vi "PXI Loop Back.vi"() -> ()   [LabVIEW 2015]
uses:
  <vilib>/Platform/TimedLoop/XDataNode/wakeup.ctl
  <vilib>/Platform/TimedLoop/XDataNode/XDNodeRunTimeDep.lvlib
  <vilib>/Platform/TimedLoop/XDataNode/nitl_modes.ctl
  <vilib>/Platform/TimedLoop/XDataNode/timing_clust.ctl
  <vilib>/Platform/TimedLoop/XDataNode/XDataNode.xnode
  <vilib>/eio/EIONode/EIONode.xnode
  <vilib>/NI Veristand/FPGA/NI_VS FPGA Support.lvlib
  <vilib>/eio/EIOMethodNode/EIOMethodNode.xnode
  <vilib>/rvi/eio/common/nirviEmuTemplateMethod_errors.vi
panel:
  in  "Enable Line":bool
  in  "ENC 2 Direction":bool
  in  "ENC 2 Periods/tic":fxp<+,32,0> format="%.32g"
  in  "ENC 1 Direction":bool
  in  "ENC 1 Periods/tic":fxp<+,32,0> format="%.32g"
  in  "ENC 0 Periods/tic":fxp<+,32,0> format="%.32g"
  in  "ENC 0 Direction":bool
  out "ENC 2 In Velocity":i32
  out "ENC 2 In Position":i32
  out "ENC 2 In Vel/Acc Update":bool
  out "ENC 1 In Velocity":i32
  out "ENC 1 In Position":i32
  out "ENC 1 In Vel/Acc Update":bool
  out "ENC 0 In Velocity":i32
  out "ENC 0 In Position":i32
  out "ENC 0 In Vel/Acc Update":bool
  in  "ENC In Clock":bool=TRUE
  in  "PWM 3 Out Low Loopback":u32
  in  "PWM 3 Out High Loopback":u32
  in  "PWM 2 Out Low Loopback":u32
  in  "PWM 2 Out High Loopback":u32
  out "PWM 1 In Low Loopback":u32
  out "PWM 1 In High Loopback":u32
  in  "PWM 1 In Timeout Loopback":u32=40000
  out "PWM 0 In Low Loopback":u32
  out "PWM 0 In High Loopback":u32
  in  "PWM 0 In Timeout Loopback":u32=40000
  out "PWM 3 In Low Time":u32
  out "PWM 3 In High Time":u32
  in  "PWM 3 In Timeout":u32=40000
  out "PWM 2 In Low Time":u32
  out "PWM 2 In High Time":u32
  in  "PWM 2 In Timeout":u32=40000
  in  "PWM 1 Out Low Time":u32
  in  "PWM 1 Out High Time":u32
  in  "PWM 0 Out Low Time":u32
  in  "PWM 0 Out High Time":u32
  in  "Generate IRQ":bool
  in  "Clock Pulse":bool
  in  "Clock Ticked":bool
  in  "Use External Timing":bool
  in  "Write to  RTSI":bool
  in  "Loop Rate (usec)":u32
  in  "Start":bool
  # "PWM out"
  # "PWM In"
  # "Encoder in"
  # "Encoder out"
  # "Configuration"
  # "Internal Controls"
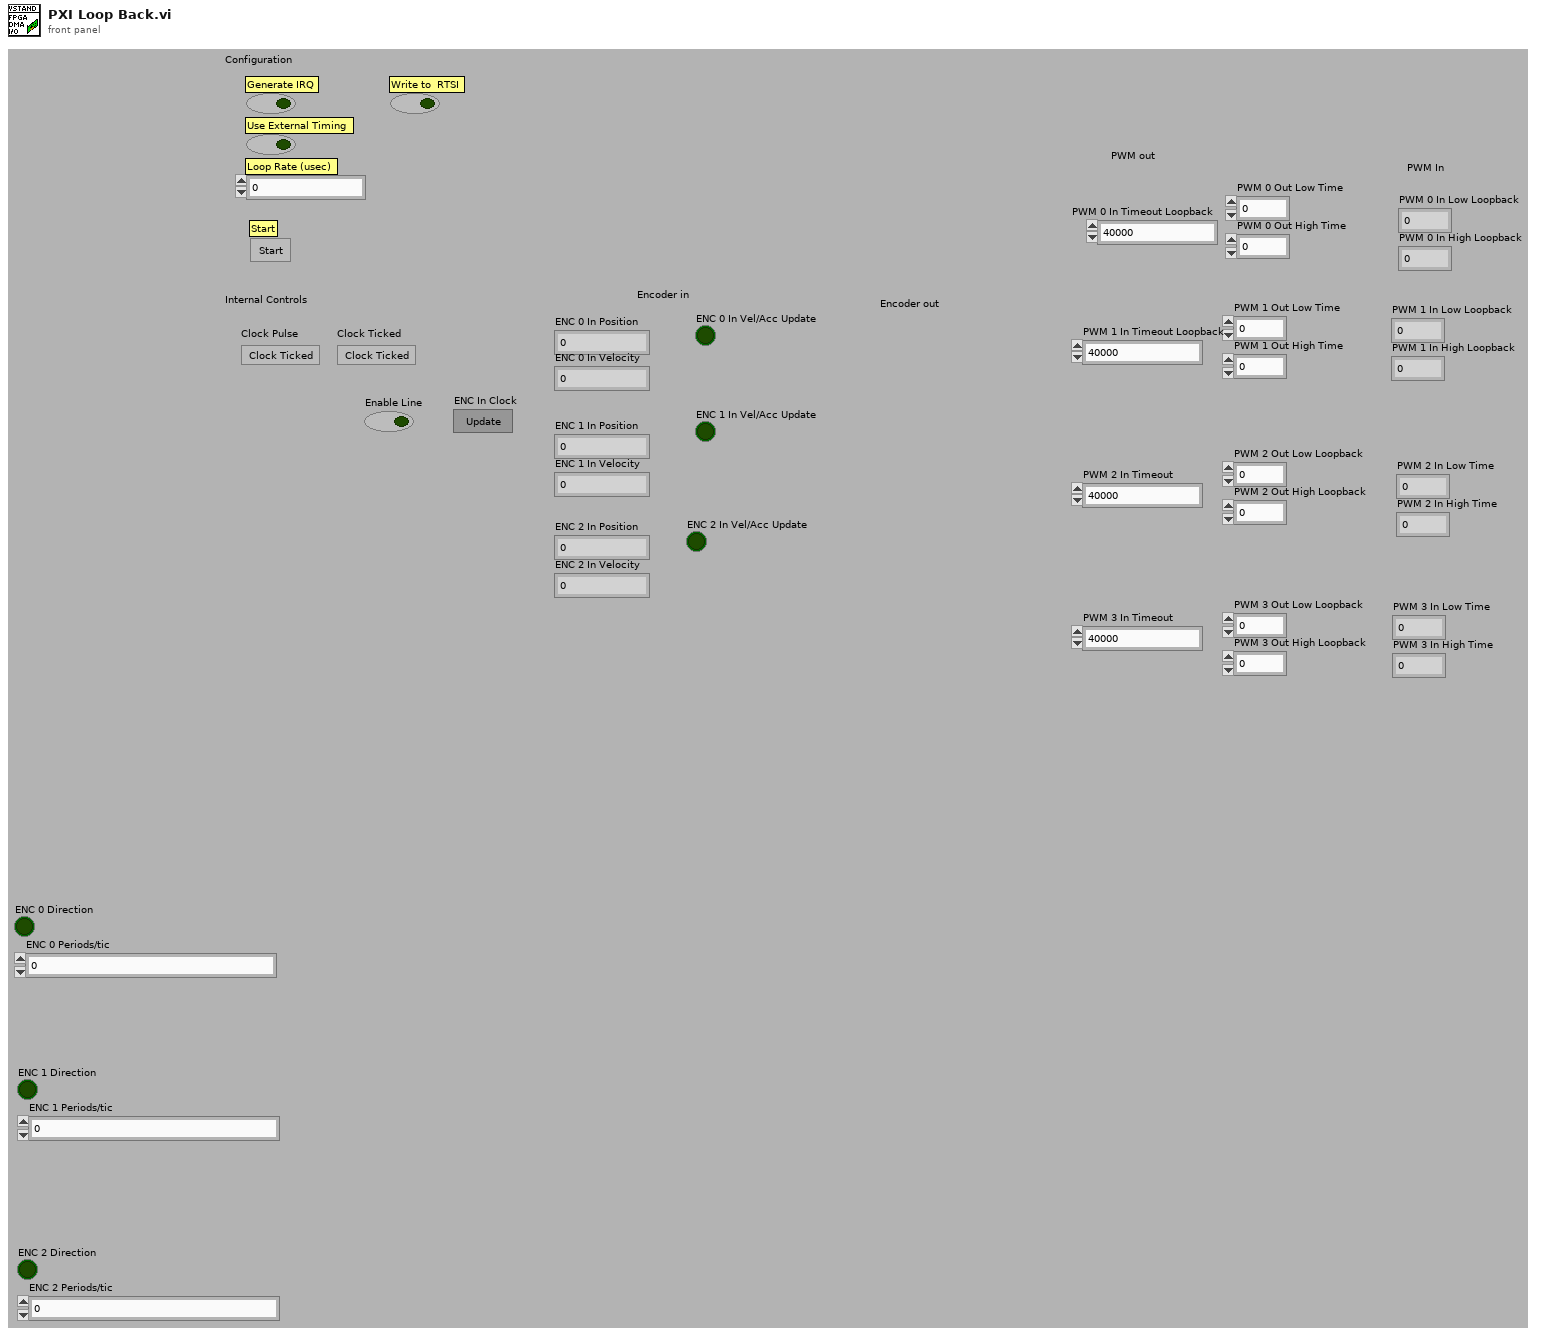
[diagram p1: front panel]
types:
  T1 = typedef "XDNodeRunTimeDep.lvlib/timing_clust.ctl" = cluster{"Expected End [f-1]":u64, "Actual End [f-1]":u64, "Finished Late? [f-1]":bool, "Expected End [i-1]":u64, "Actual End [i-1]":u64, "Finished Late? [i-1]":bool, "Expected Start [i]":u64, "Actual Start [i]":u64, "Expected Start [f]":u64, "Actual Start [f]":u64, "Source Name":string, "Structure Name":string, "Period":i64, "Deadline":i64, "Offset":i64, "Start":i64, "Priority":i32, "Timeout":i32, "Mode":T2, "Wakeup Reason":T3, "Error":errorcluster, "Source Type":string, "Secondary Source Type":string, "Global End Time":u64, "Global Start Time":u64, "Frame Duration":u64, "Iteration Duration":u64, "Assigned CPU":i32, "I/O Scan Engine Mode":u32}
  T2 = typedef "XDNodeRunTimeDep.lvlib/nitl_modes.ctl" = enum32{"No Change", "Process missed periods, maintain original phase", "Discard missed periods, maintain original phase", "Process missed periods, ignore original phase", "Discard missed periods, ignore original phase"}
  T3 = typedef "XDNodeRunTimeDep.lvlib/wakeup.ctl" = enum32{"Normal", "Aborted", "Asynchronous wakeup", "Timing source error", "Timed loop error", "Timeout"}
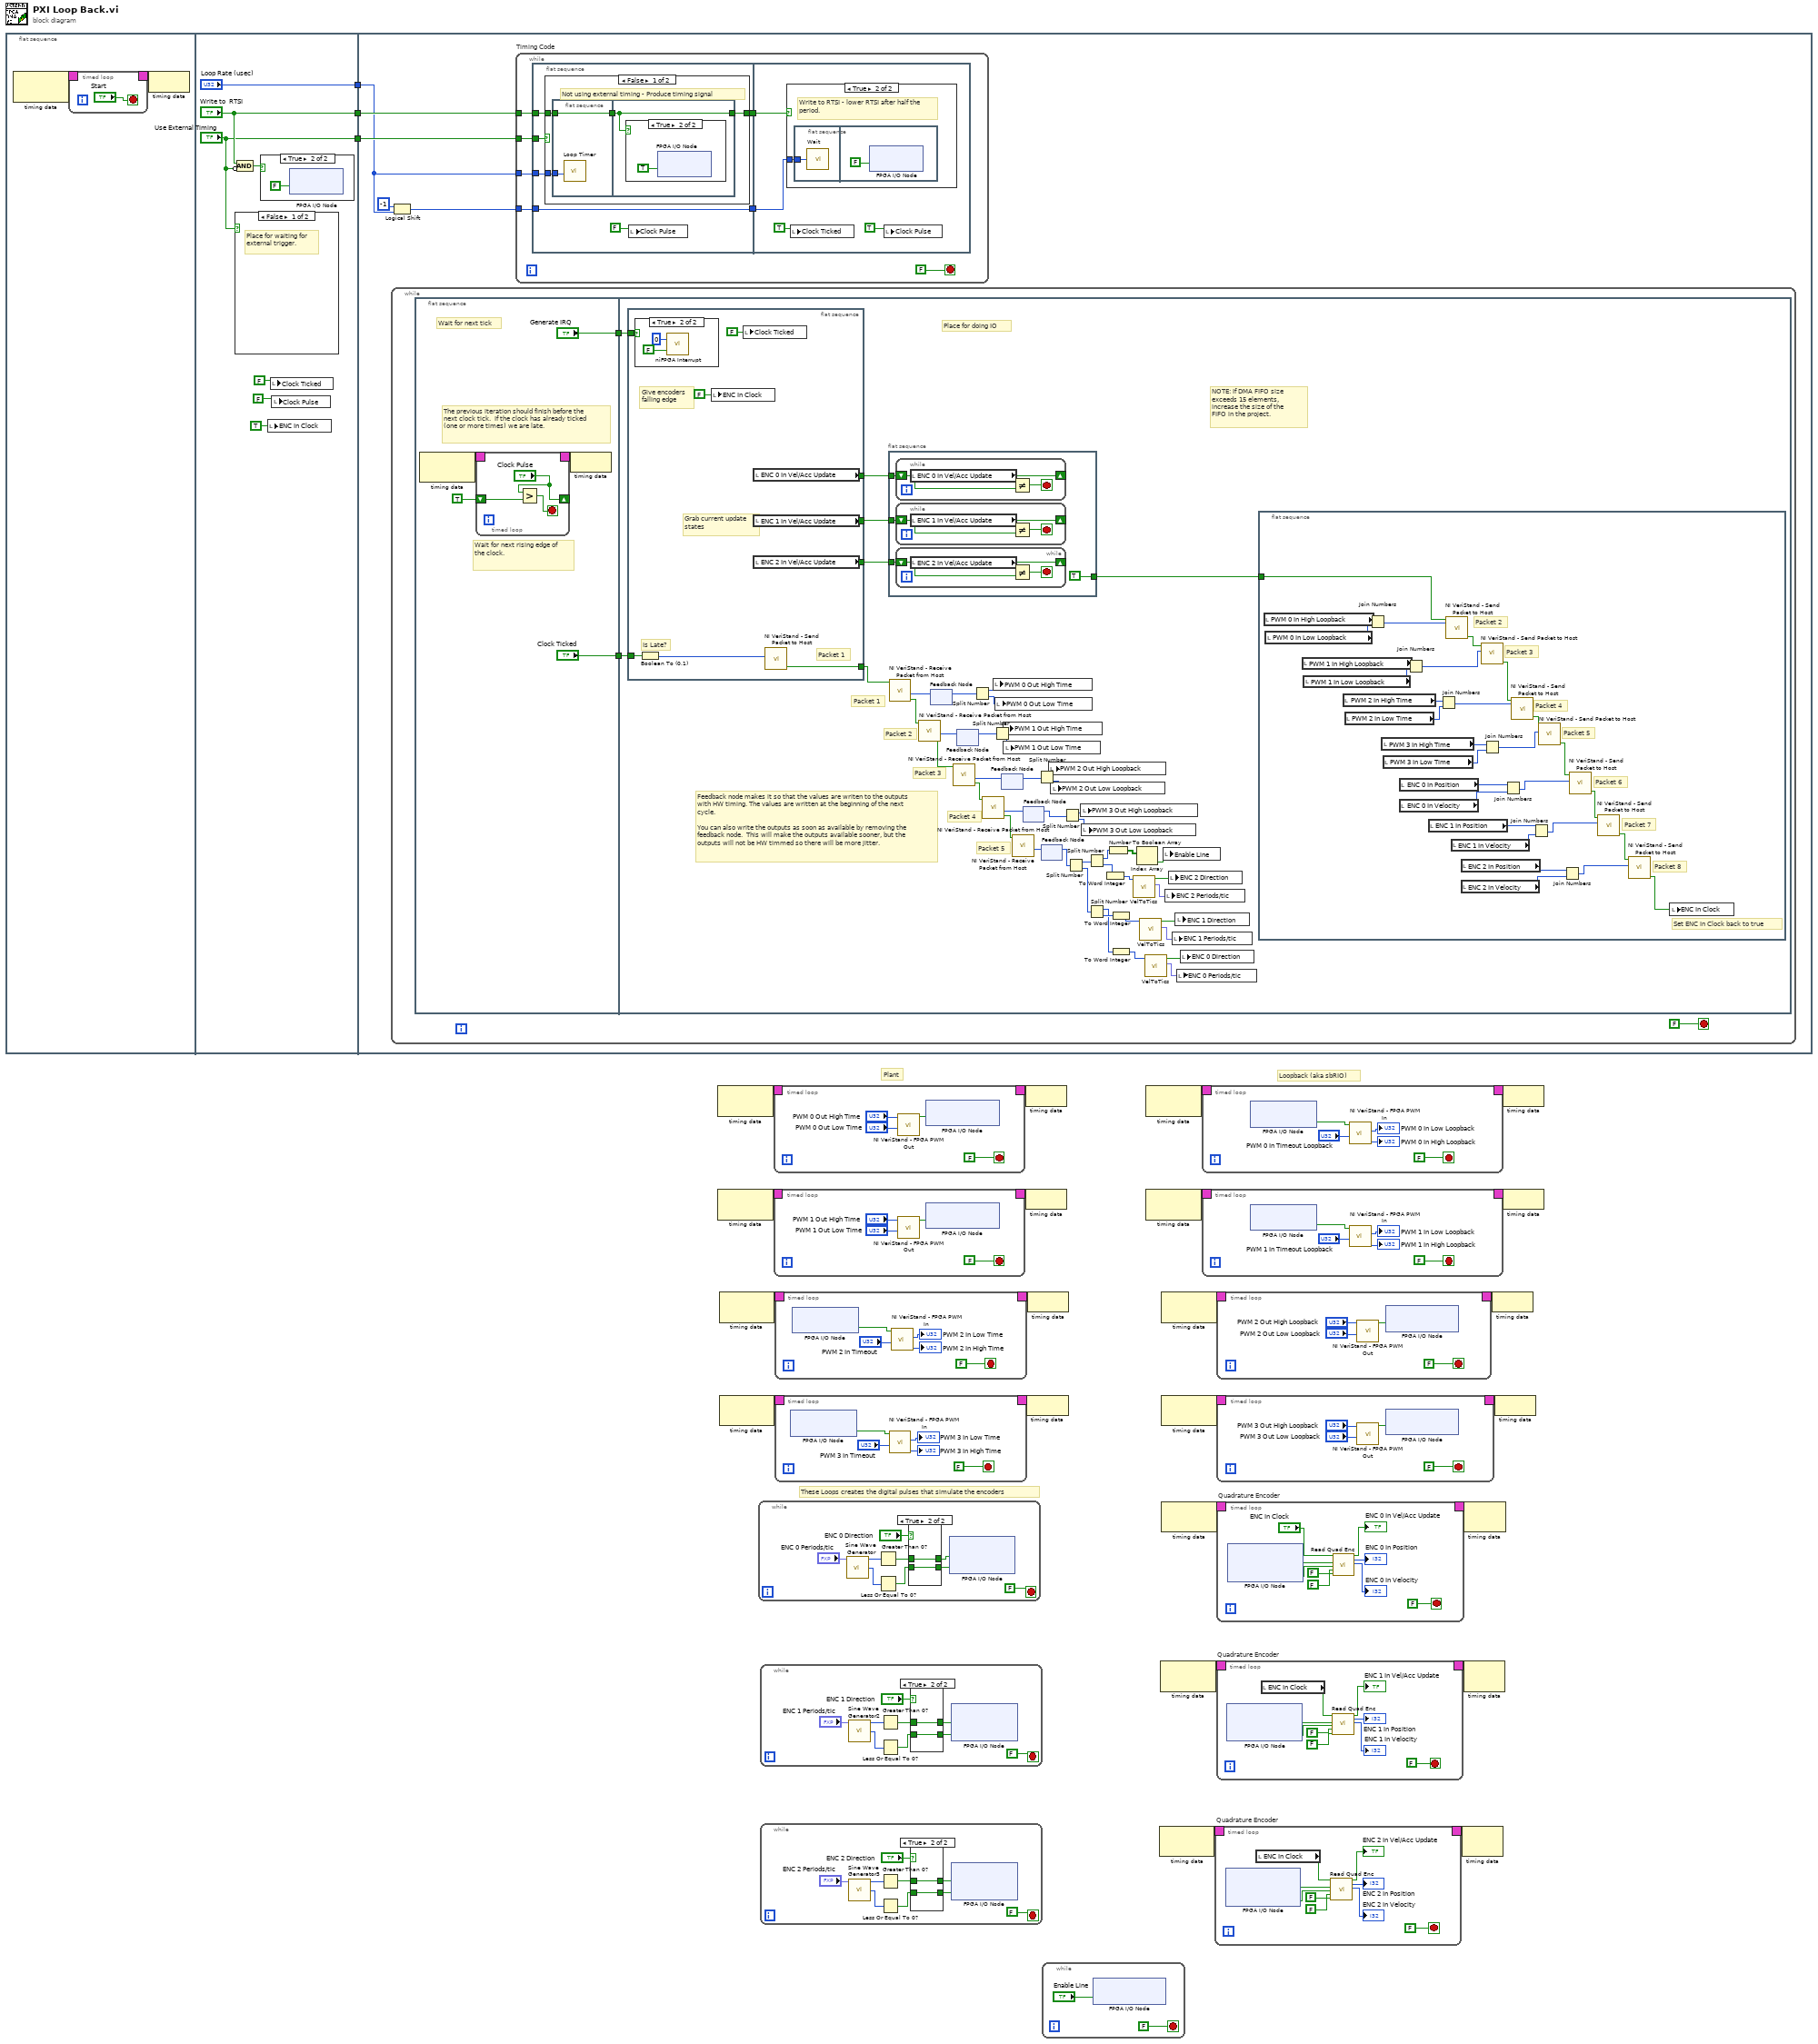
[diagram p0: block diagram]
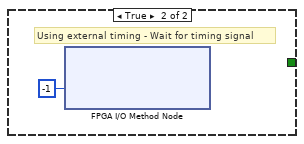
[diagram p8: hidden frame]
diagram:
  # "These Loops creates the digital pulses that simulate the encoders"
  # "Loopback (aka sbRIO)"
  # "Plant"
  n1 = flat-sequence {
    tunnel: ["Use External Timing"] -> w25
    tunnel: ["Write to  RTSI"] -> w24
    tunnel: ["Loop Rate (usec)"] -> w23
    tunnel: w25 -> [w43]
    tunnel: w24 -> [w42]
    tunnel: w23 -> [w41]
    frame #0 {
      n2 = node-c288() -> (w27:T1)  [unwired: 1 out]
      n3 = timed-loop {
        timing: w27 -> [_]
        timing-out: [_] -> w26
        stop <- "Start" stop-if-true
      }
      n4 = node-c288(w26) -> ()
    }
    frame #1 {
      n5 = case shown="False" "Use External Timing" {
        frame False {
          # "Place for waiting for external trigger."
        }
        frame True {
          # "Do not wait on trigger when externally timed."
        }
      }
      n6 = Compound Arithmetic op=AND("Write to  RTSI", invert "Use External Timing") -> (w38:bool)
      n7 = case shown="True" w38 {
        frame False {
        }
        frame True {
          n8 = xnode "FPGA I/O Node"("TRIG0"=FALSE) -> ()  [unwired: 1 in, 1 out]
        }
      }
      n9 = local write "ENC In Clock"(TRUE ("ENC In Clock")) -> ()
      n10 = local write "Clock Ticked"(FALSE ("Clock Ticked")) -> ()
      n11 = local write "Clock Pulse"(FALSE ("Clock Ticked")) -> ()
    }
    frame #2 {
      n12 = Logical Shift(y=i8 -1, x=w41) -> (x << y=w44:u32)
      n13 = while {
        stop <- FALSE stop-if-true
        n14 = flat-sequence {
          tunnel: ["Generate IRQ"] -> w76
          tunnel: ["Clock Ticked"] -> w75
          tunnel: w76 -> [w135]
          tunnel: w75 -> [w134]
          frame #0 {
            # "The previous iteration should finish before the next clock tick.  If the clock has already ticked (one or more times) we are late."
            # "Wait for next rising edge of the clock."
            # "Wait for next tick"
            n15 = node-c288() -> (w81:T1)  [unwired: 1 out]
            n16 = timed-loop {
              timing: w81 -> [_]
              timing-out: [_] -> w80
              shift-right: ["Clock Pulse"] -> _
              shift-left: TRUE ("Clock Ticked") -> [w85]
              stop <- w84 stop-if-true
              n17 = Greater?(x="Clock Pulse", y=w85) -> (0:w84:bool)
            }
            n18 = node-c288(w80) -> ()
          }
          frame #1 {
            # "Feedback node makes it so that the values are writen to the outputs with HW timing. The values are written at the beginning of the next cycle.  \n\nYou can also write the outputs as soon as available by removing the feedback node.  This will make the outputs available sooner, but the outputs will not be HW timmed so there will be more jitter."
            # "Packet 1"
            # "Packet 5"
            # "Packet 4"
            # "Packet 3"
            # "Packet 2"
            # "NOTE: If DMA FIFO size exceeds 15 elements, increase the size of the FIFO in the project."
            # "Place for doing IO"
            n19 = flat-sequence {
              tunnel: w135 -> [w186]
              tunnel: [w184] -> w108
              tunnel: w134 -> [w182]
              tunnel: [w180] -> w107
              tunnel: [w179] -> w106
              tunnel: [w178] -> w105
              frame #0 {
                # "Grab current update\nstates"
                # "Give encoders\nfalling edge"
                # "Packet 1"
                # "Is Late?"
                n20 = case shown="True" w186 {
                  frame False {
                  }
                  frame True {
                    n21 = call <vilib>:"niFPGA Interrupt.vi"("Wait Until Cleared (F)"=FALSE ("Wait Until Cleared"), "IRQ Number (0)"=u8 0 ("IRQ Number")) -> ()  [unwired: 1 in]
                  }
                }
                n22 = Boolean To (0,1)(Boolean=w182) -> (0, 1=w185:i16)
                n23 = local write "ENC In Clock"(FALSE ("ENC In Clock")) -> ()
                n24 = local write "Clock Ticked"(FALSE ("Clock Ticked")) -> ()
                n25 = local read "ENC 0 In Vel/Acc Update"() -> (w179:bool)
                n26 = local read "ENC 1 In Vel/Acc Update"() -> (w180:bool)
                n27 = local read "ENC 2 In Vel/Acc Update"() -> (w178:bool)
                n28 = call <vilib>:"NI VeriStand - Send Packet to Host.vi"("Element"=w185) -> ("Next"=w184:bool)  [unwired: 1 in, 9 out]
              }
            }
            n29 = flat-sequence {
              tunnel: w105 -> [w168]
              tunnel: w107 -> [w167]
              tunnel: w106 -> [w166]
              tunnel: [TRUE] -> w133
              frame #0 {
                n30 = while {
                  shift-right: [w170] -> _
                  shift-left: w166 -> [w171]
                  stop <- w169 stop-if-true
                  n31 = local read "ENC 0 In Vel/Acc Update"() -> (w170:bool)
                  n32 = Not Equal?(x=w170, y=w171) -> (x != y?=w169:bool)
                }
                n33 = while {
                  shift-right: [w174] -> _
                  shift-left: w167 -> [w173]
                  stop <- w172 stop-if-true
                  n34 = local read "ENC 1 In Vel/Acc Update"() -> (w174:bool)
                  n35 = Not Equal?(x=w174, y=w173) -> (x != y?=w172:bool)
                }
                n36 = while {
                  shift-right: [w176] -> _
                  shift-left: w168 -> [w177]
                  stop <- w175 stop-if-true
                  n37 = local read "ENC 2 In Vel/Acc Update"() -> (w176:bool)
                  n38 = Not Equal?(x=w176, y=w177) -> (x != y?=w175:bool)
                }
              }
            }
            n39 = call <vilib>:"NI VeriStand - Receive Packet from Host.vi"("Prev"=w108) -> ("Next"=w109:bool, "Element"=w120:u64)  [unwired: 9 in]
            n40 = call <vilib>:"NI VeriStand - Receive Packet from Host.vi"("Prev"=w109) -> ("Next"=w119:bool, "Element"=w126:u64)  [unwired: 9 in]
            n41 = feedback-in #1(w120) -> ()
            n42 = feedback #1() -> (w121:u64)  [unwired: 1 in]
            n43 = call <vilib>:"NI VeriStand - Receive Packet from Host.vi"("Prev"=w119) -> ("Next"=w118:bool, "Element"=w124:u64)  [unwired: 9 in]
            n44 = feedback-in #2(w126) -> ()
            n45 = feedback #2() -> (w127:u64)  [unwired: 1 in]
            n46 = Split Number(x=w121) -> (hi(x)=w111:u32, lo(x)=w110:u32)
            n47 = call <vilib>:"NI VeriStand - Receive Packet from Host.vi"("Prev"=w118) -> ("Next"=w128:bool, "Element"=w122:u64)  [unwired: 9 in]
            n48 = Split Number(x=w127) -> (hi(x)=w112:u32, lo(x)=w113:u32)
            n49 = local write "PWM 0 Out High Time"(w111) -> ()
            n50 = local write "PWM 0 Out Low Time"(w110) -> ()
            n51 = feedback-in #3(w124) -> ()
            n52 = feedback #3() -> (w125:u64)  [unwired: 1 in]
            n53 = local write "PWM 1 Out High Time"(w112) -> ()
            n54 = local write "PWM 1 Out Low Time"(w113) -> ()
            n55 = call <vilib>:"NI VeriStand - Receive Packet from Host.vi"("Prev"=w128) -> ("Element"=w129:u64)  [unwired: 9 in, 1 out]
            n56 = feedback-in #4(w122) -> ()
            n57 = feedback #4() -> (w123:u64)  [unwired: 1 in]
            n58 = Split Number(x=w125) -> (hi(x)=w116:u32, lo(x)=w117:u32)
            n59 = feedback-in #5(w129) -> ()
            n60 = feedback #5() -> (w130:u64)  [unwired: 1 in]
            n61 = local write "PWM 2 Out High Loopback"(w116) -> ()
            n62 = local write "PWM 2 Out Low Loopback"(w117) -> ()
            n63 = Split Number(x=w123) -> (hi(x)=w115:u32, lo(x)=w114:u32)
            n64 = Split Number(x=w130) -> (hi(x)=w131:u32, lo(x)=w132:u32)
            n65 = local write "PWM 3 Out High Loopback"(w115) -> ()
            n66 = local write "PWM 3 Out Low Loopback"(w114) -> ()
            n67 = Split Number(x=w131) -> (hi(x)=w92:u16, lo(x)=w104:u16)
            n68 = Split Number(x=w132) -> (hi(x)=w103:u16, lo(x)=w102:u16)
            n69 = To Word Integer(number=w104) -> (16bit integer=w101:i16)
            n70 = Number To Boolean Array(number=w92) -> (Boolean array=w91:bool[])
            n71 = To Word Integer(number=w103) -> (16bit integer=w94:i16)
            n72 = To Word Integer(number=w102) -> (16bit integer=w93:i16)
            n73 = call "VelToTics.vi"("Velocity/Sec"=w101) -> ("Periods/tic"=w99:fxp<+,32,0>, "Direction"=w100:bool)  [unwired: 9 in]
            n74 = Index Array(array=w91) -> (element=w90:bool)  [unwired: 1 in]
            n75 = call "VelToTics.vi"("Velocity/Sec"=w94) -> ("Periods/tic"=w98:fxp<+,32,0>, "Direction"=w97:bool)  [unwired: 9 in]
            n76 = call "VelToTics.vi"("Velocity/Sec"=w93) -> ("Periods/tic"=w95:fxp<+,32,0>, "Direction"=w96:bool)  [unwired: 9 in]
            n77 = local write "Enable Line"(w90) -> ()
            n78 = local write "ENC 2 Periods/tic"(w99) -> ()
            n79 = local write "ENC 2 Direction"(w100) -> ()
            n80 = local write "ENC 1 Periods/tic"(w98) -> ()
            n81 = local write "ENC 1 Direction"(w97) -> ()
            n82 = local write "ENC 0 Periods/tic"(w95) -> ()
            n83 = local write "ENC 0 Direction"(w96) -> ()
            n84 = flat-sequence {
              tunnel: w133 -> [w159]
              frame #0 {
                # "Set ENC In Clock back to true"
                # "Packet 8"
                # "Packet 7"
                # "Packet 6"
                # "Packet 5"
                # "Packet 3"
                # "Packet 4"
                # "Packet 2"
                n85 = local read "PWM 0 In High Loopback"() -> (w142:u32)
                n86 = local read "PWM 0 In Low Loopback"() -> (w141:u32)
                n87 = local read "PWM 1 In High Loopback"() -> (w137:u32)
                n88 = local read "PWM 1 In Low Loopback"() -> (w138:u32)
                n89 = local read "PWM 2 In High Time"() -> (w143:u32)
                n90 = local read "PWM 2 In Low Time"() -> (w144:u32)
                n91 = Join Numbers(hi=w142, lo=w141) -> ((hi.lo)=w140:u64)
                n92 = local read "PWM 3 In High Time"() -> (w148:u32)
                n93 = local read "PWM 3 In Low Time"() -> (w147:u32)
                n94 = local read "ENC 0 In Position"() -> (w152:i32)
                n95 = local read "ENC 0 In Velocity"() -> (w153:i32)
                n96 = Join Numbers(hi=w137, lo=w138) -> ((hi.lo)=w136:u64)
                n97 = local read "ENC 1 In Position"() -> (w160:i32)
                n98 = Join Numbers(hi=w143, lo=w144) -> ((hi.lo)=w145:u64)
                n99 = call <vilib>:"NI VeriStand - Send Packet to Host.vi"("Element"=w140, "Prev"=w159) -> ("Next"=w139:bool)  [unwired: 9 in]
                n100 = local read "ENC 1 In Velocity"() -> (w161:i32)
                n101 = local read "ENC 2 In Position"() -> (w162:i32)
                n102 = local read "ENC 2 In Velocity"() -> (w163:i32)
                n103 = call <vilib>:"NI VeriStand - Send Packet to Host.vi"("Element"=w136, "Prev"=w139) -> ("Next"=w150:bool)  [unwired: 9 in]
                n104 = Join Numbers(hi=w148, lo=w147) -> ((hi.lo)=w149:u64)
                n105 = Join Numbers(hi=w152, lo=w153) -> ((hi.lo)=w154:u64)
                n106 = call <vilib>:"NI VeriStand - Send Packet to Host.vi"("Element"=w145, "Prev"=w150) -> ("Next"=w146:bool)  [unwired: 9 in]
                n107 = Join Numbers(hi=w160, lo=w161) -> ((hi.lo)=w155:u64)
                n108 = call <vilib>:"NI VeriStand - Send Packet to Host.vi"("Element"=w149, "Prev"=w146) -> ("Next"=w151:bool)  [unwired: 9 in]
                n109 = Join Numbers(hi=w162, lo=w163) -> ((hi.lo)=w156:u64)
                n110 = call <vilib>:"NI VeriStand - Send Packet to Host.vi"("Element"=w154, "Prev"=w151) -> ("Next"=w158:bool)  [unwired: 9 in]
                n111 = call <vilib>:"NI VeriStand - Send Packet to Host.vi"("Element"=w155, "Prev"=w158) -> ("Next"=w157:bool)  [unwired: 9 in]
                n112 = call <vilib>:"NI VeriStand - Send Packet to Host.vi"("Element"=w156, "Prev"=w157) -> ("Next"=w164:bool)  [unwired: 9 in]
                n113 = local write "ENC In Clock"(w164) -> ()
              }
            }
          }
        }
      }
      n114 = while "Timing Code" {
        tunnel: w44 -> [w52]
        tunnel: w41 -> [w51]
        tunnel: w43 -> [w50]
        tunnel: w42 -> [w49]
        stop <- FALSE stop-if-true
        n115 = flat-sequence {
          tunnel: w52 -> [w55]
          tunnel: w51 -> [w58]
          tunnel: w50 -> [w57]
          tunnel: w49 -> [w56]
          tunnel: [w55] -> w47
          tunnel: [w53] -> w46
          tunnel: w47 -> [w71]
          tunnel: w46 -> [w68]
          frame #0 {
            n116 = case shown="False" w57 {
              tunnel: w58 -> [w62 _]
              tunnel: w56 -> [w60 _]
              tunnel: [w59 _] -> w53
              frame False {
                # "Not using external timing - Produce timing signal"
                n117 = flat-sequence {
                  tunnel: [w63] -> w61
                  tunnel: w62 -> [w64]
                  tunnel: w60 -> [w63]
                  tunnel: w61 -> [w65]
                  tunnel: [w65] -> w59
                  frame #0 {
                    n118 = call "Loop Timer"("Count(uSec)"=w64) -> ()  [unwired: 1 out]
                  }
                  frame #1 {
                    n119 = case shown="True" w65 {
                      frame False {
                      }
                      frame True {
                        n120 = xnode "FPGA I/O Node"("TRIG0"=TRUE) -> ()  [unwired: 1 in, 1 out]
                      }
                    }
                  }
                }
              }
              frame True {
                # "Using external timing - Wait for timing signal"
                n121 = xnode "FPGA I/O Method Node"("Timeout"=-1) -> ()  [unwired: 1 in, 2 out]
              }
            }
            n122 = local write "Clock Pulse"(FALSE ("Clock Ticked")) -> ()
          }
          frame #1 {
            n123 = case shown="True" w68 {
              tunnel: w71 -> [_ w72]
              frame False {
              }
              frame True {
                # "Write to RTSI - lower RTSI after half the period."
                n124 = flat-sequence {
                  tunnel: w72 -> [w73]
                  frame #0 {
                    n125 = call "Wait"("Count(uSec)"=w73) -> ()  [unwired: 1 out]
                  }
                  frame #1 {
                    n126 = xnode "FPGA I/O Node"("TRIG0"=FALSE) -> ()  [unwired: 1 in, 1 out]
                  }
                }
              }
            }
            n127 = local write "Clock Ticked"(TRUE ("Clock Ticked")) -> ()
            n128 = local write "Clock Pulse"(TRUE ("Clock Ticked")) -> ()
          }
        }
      }
    }
  }
  n129 = node-c288() -> (w22:T1)  [unwired: 1 in]
  n130 = node-c288() -> (w20:T1)  [unwired: 1 in]
  n131 = node-c288() -> (w18:T1)  [unwired: 1 in]
  n132 = node-c288() -> (w16:T1)  [unwired: 1 in]
  n133 = while {
    stop <- FALSE stop-if-true
    n134 = call "Sine Wave Generator"("frequency (periods/tick)"="ENC 0 Periods/tic") -> ("sine out"=w196:i8, "cosine out"=w195:i8)  [unwired: 13 in]
    n135 = Greater Than 0?(x=w196) -> (x > 0?=w192:bool)
    n136 = Less Or Equal To 0?(x=w195) -> (x <= 0?=w190:bool)
    n137 = case shown="True" "ENC 0 Direction" {
      tunnel: [w198 w201] -> w191
      tunnel: w192 -> [w199 w201]
      tunnel: [w199 w200] -> w189
      tunnel: w190 -> [w198 w200]
      frame False {
      }
      frame True {
      }
    }
    n138 = xnode "FPGA I/O Node"("ENC 0 A+"=w191, "ENC 0 B+"=w189) -> ()  [unwired: 2 in, 2 out]
  }
  n139 = while {
    stop <- FALSE stop-if-true
    n140 = call "Sine Wave Generator2"("frequency (periods/tick)"="ENC 1 Periods/tic") -> ("sine out"=w209:i8, "cosine out"=w208:i8)  [unwired: 13 in]
    n141 = Greater Than 0?(x=w209) -> (x > 0?=w205:bool)
    n142 = Less Or Equal To 0?(x=w208) -> (x <= 0?=w203:bool)
    n143 = case shown="True" "ENC 1 Direction" {
      tunnel: [w211 w214] -> w204
      tunnel: w205 -> [w212 w214]
      tunnel: [w212 w213] -> w202
      tunnel: w203 -> [w211 w213]
      frame False {
      }
      frame True {
      }
    }
    n144 = xnode "FPGA I/O Node"("ENC 1 A+"=w204, "ENC 1 B+"=w202) -> ()  [unwired: 2 in, 2 out]
  }
  n145 = while {
    stop <- FALSE stop-if-true
    n146 = call "Sine Wave Generator3"("frequency (periods/tick)"="ENC 2 Periods/tic") -> ("sine out"=w222:i8, "cosine out"=w221:i8)  [unwired: 13 in]
    n147 = Greater Than 0?(x=w222) -> (x > 0?=w218:bool)
    n148 = Less Or Equal To 0?(x=w221) -> (x <= 0?=w216:bool)
    n149 = case shown="True" "ENC 2 Direction" {
      tunnel: [w224 w227] -> w217
      tunnel: w218 -> [w225 w227]
      tunnel: [w225 w226] -> w215
      tunnel: w216 -> [w224 w226]
      frame False {
      }
      frame True {
      }
    }
    n150 = xnode "FPGA I/O Node"("ENC 2 A+"=w217, "ENC 2 B+"=w215) -> ()  [unwired: 2 in, 2 out]
  }
  n151 = timed-loop {
    timing: w22 -> [_]
    timing-out: [_] -> w21
    stop <- FALSE stop-if-true
    n152 = call <vilib>:"NI VeriStand - FPGA PWM Out.vi"("_Low Time"="PWM 0 Out Low Time", "_High Time"="PWM 0 Out High Time") -> ("Output"=w228:bool)  [unwired: 9 in]
    n153 = xnode "FPGA I/O Node"("PWM 0 Out"=w228) -> ()  [unwired: 1 in, 1 out]
  }
  n154 = timed-loop {
    timing: w20 -> [_]
    timing-out: [_] -> w19
    stop <- FALSE stop-if-true
    n155 = call <vilib>:"NI VeriStand - FPGA PWM Out.vi"("_Low Time"="PWM 1 Out Low Time", "_High Time"="PWM 1 Out High Time") -> ("Output"=w234:bool)  [unwired: 9 in]
    n156 = xnode "FPGA I/O Node"("PWM 1 Out"=w234) -> ()  [unwired: 1 in, 1 out]
  }
  n157 = timed-loop {
    timing: w18 -> [_]
    timing-out: [_] -> w17
    stop <- FALSE stop-if-true
    n158 = xnode "FPGA I/O Node"() -> ("PWM 2 In"=w243:bool)  [unwired: 1 in, 1 out]
    n159 = call <vilib>:"NI VeriStand - FPGA PWM In.vi"("Time Out"="PWM 2 In Timeout", "Value"=w243) -> ("High time"=→"PWM 2 In High Time":u32, "Low Time"=→"PWM 2 In Low Time":u32)  [unwired: 8 in]
  }
  n160 = timed-loop {
    timing: w16 -> [_]
    timing-out: [_] -> w15
    stop <- FALSE stop-if-true
    n161 = xnode "FPGA I/O Node"() -> ("PWM 3 In"=w250:bool)  [unwired: 1 in, 1 out]
    n162 = call <vilib>:"NI VeriStand - FPGA PWM In.vi"("Time Out"="PWM 3 In Timeout", "Value"=w250) -> ("High time"=→"PWM 3 In High Time":u32, "Low Time"=→"PWM 3 In Low Time":u32)  [unwired: 8 in]
  }
  n163 = node-c288(w21) -> ()
  n164 = node-c288(w19) -> ()
  n165 = node-c288(w15) -> ()
  n166 = node-c288(w17) -> ()
  n167 = while {
    stop <- FALSE stop-if-true
    n168 = xnode "FPGA I/O Node"("Enable Line"="Enable Line") -> ()  [unwired: 1 in, 1 out]
  }
  n169 = node-c288() -> (w14:T1)  [unwired: 1 in]
  n170 = node-c288() -> (w12:T1)  [unwired: 1 in]
  n171 = node-c288() -> (w2:T1)  [unwired: 1 in]
  n172 = node-c288() -> (w4:T1)  [unwired: 1 in]
  n173 = node-c288() -> (w10:T1)  [unwired: 1 in]
  n174 = node-c288() -> (w8:T1)  [unwired: 1 in]
  n175 = node-c288() -> (w6:T1)  [unwired: 1 in]
  n176 = timed-loop {
    timing: w14 -> [_]
    timing-out: [_] -> w13
    stop <- FALSE stop-if-true
    n177 = xnode "FPGA I/O Node"() -> ("PWM 0 In"=w259:bool)  [unwired: 1 in, 1 out]
    n178 = call <vilib>:"NI VeriStand - FPGA PWM In.vi"("Time Out"="PWM 0 In Timeout Loopback", "Value"=w259) -> ("High time"=→"PWM 0 In High Loopback":u32, "Low Time"=→"PWM 0 In Low Loopback":u32)  [unwired: 8 in]
  }
  n179 = timed-loop {
    timing: w12 -> [_]
    timing-out: [_] -> w11
    stop <- FALSE stop-if-true
    n180 = xnode "FPGA I/O Node"() -> ("PWM 1 In"=w266:bool)  [unwired: 1 in, 1 out]
    n181 = call <vilib>:"NI VeriStand - FPGA PWM In.vi"("Time Out"="PWM 1 In Timeout Loopback", "Value"=w266) -> ("High time"=→"PWM 1 In High Loopback":u32, "Low Time"=→"PWM 1 In Low Loopback":u32)  [unwired: 8 in]
  }
  n182 = timed-loop "Quadrature Encoder" {
    timing: w2 -> [_]
    timing-out: [_] -> w1
    stop <- FALSE ("stop") stop-if-true
    n183 = xnode "FPGA I/O Node"() -> ("ENC 2 A+ In"=w273:bool, "ENC 2 B+ In"=w272:bool)  [unwired: 2 in, 2 out]
    n184 = local read "ENC In Clock"() -> (w270:bool)
    n185 = call "Read Quad Enc.vi"("Clock"=w270, "A"=w273, "B"=w272, "Z"=FALSE, "Polarity"=FALSE) -> ("Vel/Acc Update"=→"ENC 2 In Vel/Acc Update":bool, "Position (Counts)"=→"ENC 2 In Position":i32, "Velocity (Counts/Interval)"=→"ENC 2 In Velocity":i32)  [unwired: 3 in, 9 out]
  }
  n186 = timed-loop "Quadrature Encoder" {
    timing: w4 -> [_]
    timing-out: [_] -> w3
    stop <- FALSE ("stop") stop-if-true
    n187 = xnode "FPGA I/O Node"() -> ("ENC 1 A+ In"=w284:bool, "ENC 1 B+ In"=w283:bool)  [unwired: 2 in, 2 out]
    n188 = local read "ENC In Clock"() -> (w281:bool)
    n189 = call "Read Quad Enc.vi"("Clock"=w281, "A"=w284, "B"=w283, "Z"=FALSE, "Polarity"=FALSE) -> ("Vel/Acc Update"=→"ENC 1 In Vel/Acc Update":bool, "Position (Counts)"=→"ENC 1 In Position":i32, "Velocity (Counts/Interval)"=→"ENC 1 In Velocity":i32)  [unwired: 3 in, 9 out]
  }
  n190 = timed-loop {
    timing: w10 -> [_]
    timing-out: [_] -> w9
    stop <- FALSE stop-if-true
    n191 = call <vilib>:"NI VeriStand - FPGA PWM Out.vi"("_Low Time"="PWM 2 Out Low Loopback", "_High Time"="PWM 2 Out High Loopback") -> ("Output"=w292:bool)  [unwired: 9 in]
    n192 = xnode "FPGA I/O Node"("PWM 2 Out"=w292) -> ()  [unwired: 1 in, 1 out]
  }
  n193 = timed-loop {
    timing: w8 -> [_]
    timing-out: [_] -> w7
    stop <- FALSE stop-if-true
    n194 = call <vilib>:"NI VeriStand - FPGA PWM Out.vi"("_Low Time"="PWM 3 Out Low Loopback", "_High Time"="PWM 3 Out High Loopback") -> ("Output"=w298:bool)  [unwired: 9 in]
    n195 = xnode "FPGA I/O Node"("PWM 3 Out"=w298) -> ()  [unwired: 1 in, 1 out]
  }
  n196 = timed-loop "Quadrature Encoder" {
    timing: w6 -> [_]
    timing-out: [_] -> w5
    stop <- FALSE ("stop") stop-if-true
    n197 = xnode "FPGA I/O Node"() -> ("ENC 0 A+ In"=w307:bool, "ENC 0 B+ In"=w306:bool)  [unwired: 2 in, 2 out]
    n198 = call "Read Quad Enc.vi"("Clock"="ENC In Clock", "A"=w307, "B"=w306, "Z"=FALSE, "Polarity"=FALSE) -> ("Vel/Acc Update"=→"ENC 0 In Vel/Acc Update":bool, "Position (Counts)"=→"ENC 0 In Position":i32, "Velocity (Counts/Interval)"=→"ENC 0 In Velocity":i32)  [unwired: 3 in, 9 out]
  }
  n199 = node-c288(w1) -> ()  [unwired: 1 out]
  n200 = node-c288(w3) -> ()  [unwired: 1 out]
  n201 = node-c288(w5) -> ()  [unwired: 1 out]
  n202 = node-c288(w9) -> ()
  n203 = node-c288(w7) -> ()
  n204 = node-c288(w13) -> ()
  n205 = node-c288(w11) -> ()
